vi "Write Position.vi"(8 "error in (no error)":errorcluster, 10 "position":T1, 11 "Velodyne 3D LIDAR in":refnum<class "Velodyne 3D LIDAR.lvclass">) -> (0 "error out":errorcluster, 3 "Velodyne 3D LIDAR out":refnum<class "Velodyne 3D LIDAR.lvclass">)   [LabVIEW 2017, in "NI_Robotics_Simulator.lvlib" / "Velodyne 3D LIDAR.lvclass"]
uses:
  <vilib>/robotics/Simulator/Plugin/Sensor/Velodyne 3D LIDAR/Velodyne 3D LIDAR.lvclass
  <vilib>/Utility/miscctls.llb/LV3DPointTypeDef.ctl
  <vilib>/robotics/Simulator/Plugin/Sensor/Velodyne 3D LIDAR/Velodyne 3D LIDAR.lvclass/Velodyne 3D LIDAR.ctl
  <vilib>/robotics/Simulator/Robot Factory/Sensor/Base/ODESimulator_Base_Sensor.lvclass
  <vilib>/robotics/Simulator/3D-Physics/Sphere/3D_Physics_Sphere.lvclass
  <vilib>/robotics/Simulator/Robot Factory/Sensor/LIDAR/ODESimulator_LIDAR.lvclass
  <vilib>/robotics/Simulator/Robot Factory/Joint/ODESimulator_Joint.lvclass
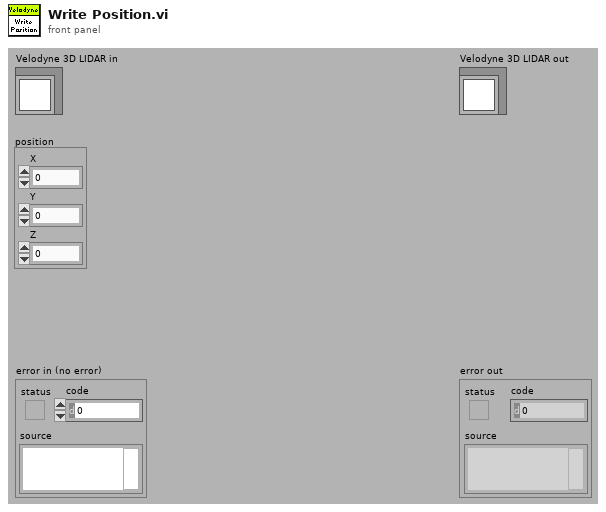
[diagram p1: front panel]
types:
  T1 = typedef "LV3DPointTypeDef.ctl" = cluster{"X":sgl, "Y":sgl, "Z":sgl}
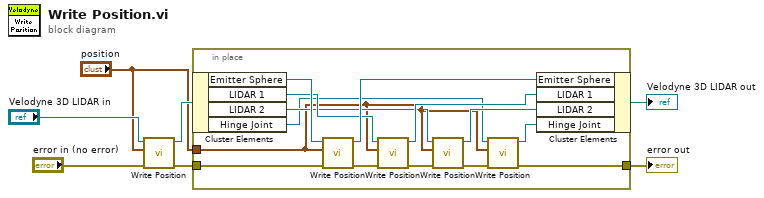
[diagram p0: block diagram]
diagram:
  n1 = call-parent <vilib>:"Write Position.vi"("error in (no error)"="error in (no error)", "position"="position", "ODESimulator_Base_Sensor in"="Velodyne 3D LIDAR in") -> ("error out"=w3:errorcluster, "ODESimulator_Base_Sensor out"=w5:refnum<class "Velodyne 3D LIDAR.lvclass">)  [unwired: 7 in]
  n2 = in-place {
    in-place-border: "position" -> [w11]
    in-place-border: w3 -> [w20]
    in-place-border: [w9] -> w2
    n3 = in-place-cluster #1(w5) -> ("Emitter Sphere"=w21:refnum<class "3D_Physics_Sphere.lvclass">, "LIDAR 1"=w18:refnum<class "ODESimulator_LIDAR.lvclass">, "LIDAR 2"=w14:refnum<class "ODESimulator_LIDAR.lvclass">, "Hinge Joint"=w12:refnum<class "ODESimulator_Joint.lvclass">)
    n4 = call-dynamic <vilib>:"Write Position.vi"("error in (no error)"=w20, "3D Point"=w11, "Base in"=w21) -> ("error out"=w17:errorcluster, "Base out"=w19:refnum<class "3D_Physics_Sphere.lvclass">)  [unwired: 7 in]
    n5 = call-dynamic <vilib>:"Write Position.vi"("error in (no error)"=w17, "position"=w11, "ODESimulator_Base_Sensor in"=w18) -> ("error out"=w16:errorcluster, "ODESimulator_Base_Sensor out"=w15:refnum<class "ODESimulator_LIDAR.lvclass">)  [unwired: 7 in]
    n6 = call-dynamic <vilib>:"Write Position.vi"("error in (no error)"=w16, "position"=w11, "ODESimulator_Base_Sensor in"=w14) -> ("error out"=w10:errorcluster, "ODESimulator_Base_Sensor out"=w13:refnum<class "ODESimulator_LIDAR.lvclass">)  [unwired: 7 in]
    n7 = call <vilib>:"Write Position.vi"("error in (no error)"=w10, "3D Point"=w11, "ODESimulator_Joint in"=w12) -> ("error out"=w9:errorcluster, "ODESimulator_Joint out"=w8:refnum<class "ODESimulator_Joint.lvclass">)  [unwired: 7 in]
    n8 = in-place-cluster #1("Emitter Sphere"=w19, "LIDAR 1"=w15, "LIDAR 2"=w13, "Hinge Joint"=w8) -> (→"Velodyne 3D LIDAR out":refnum<class "Velodyne 3D LIDAR.lvclass">)
  }
  "error out" <- w2
